vi "Main.vi"() -> ()   [LabVIEW 2020]
uses:
  Ctrl/Ctrl_state_FGV.ctl
panel:
  out "Read Data":u8
  in  "Commande":T1
  out "Compteur 4":dbl
  out "Compteur 3":dbl
  out "Compteur 2":dbl
  out "Compteur":dbl
  # "Non re-entrant"
  # "re-entrant"
  # "FGV"
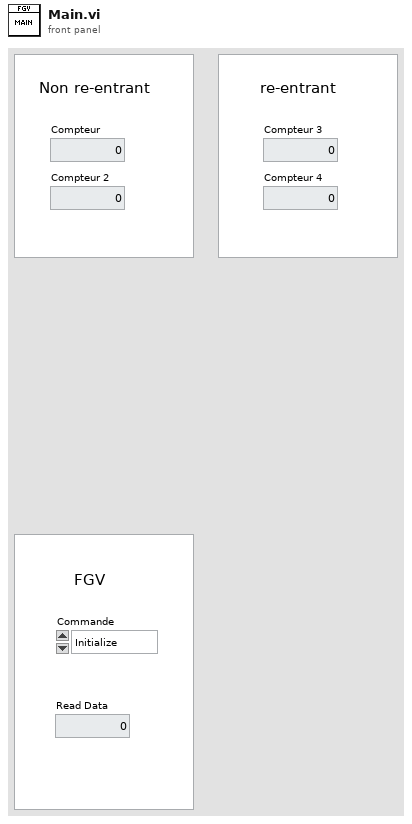
[diagram p1: front panel]
types:
  T1 = typedef "Ctrl_state_FGV.ctl" = enum16{"Initialize", "Write", "Read"}
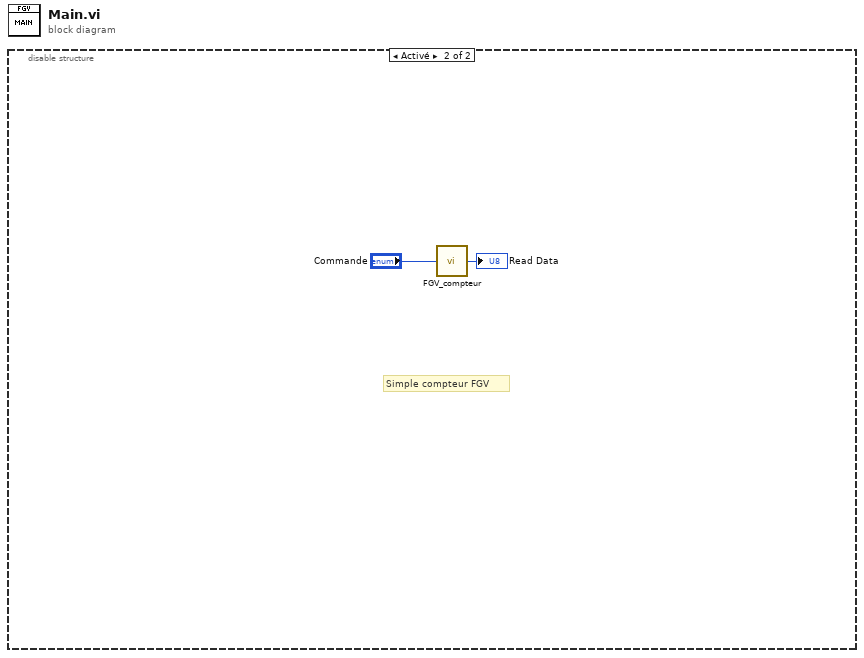
[diagram p0: block diagram]
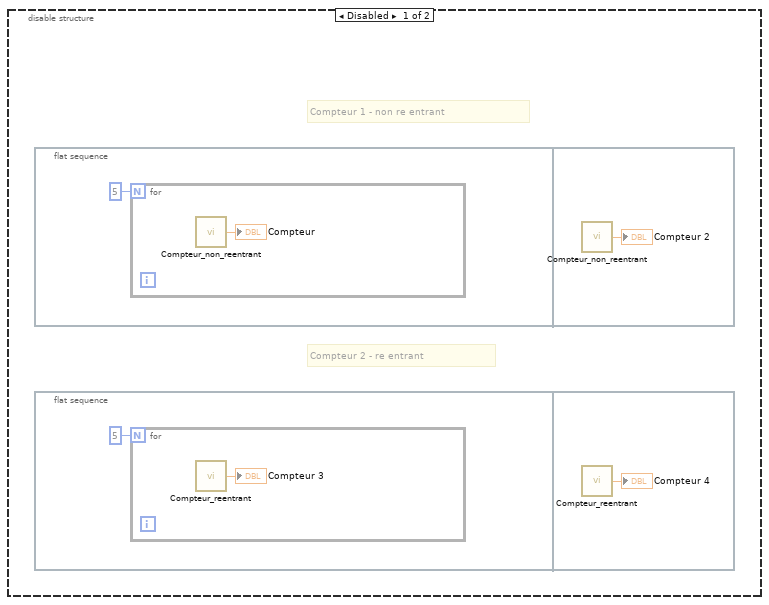
[diagram p2: hidden frame]
diagram:
  n1 = disable-structure shown="Activé" {
    frame Disabled {
      # "Compteur 2 - re entrant"
      # "Compteur 1 - non re entrant"
      n2 = flat-sequence {
        frame #0 {
          n3 = for {
            N: 5 -> [_]
            n4 = call "Compteur_non_reentrant.vi"() -> ("Compteur"=→"Compteur":dbl)  [unwired: 1 in]
          }
        }
        frame #1 {
          n5 = call "Compteur_non_reentrant.vi"() -> ("Compteur"=→"Compteur 2":dbl)  [unwired: 1 in]
        }
      }
      n6 = flat-sequence {
        frame #0 {
          n7 = for {
            N: 5 -> [_]
            n8 = call "Compteur_reentrant.vi"() -> ("Compteur"=→"Compteur 3":dbl)  [unwired: 1 in]
          }
        }
        frame #1 {
          n9 = call "Compteur_reentrant.vi"() -> ("Compteur"=→"Compteur 4":dbl)  [unwired: 1 in]
        }
      }
    }
    frame Enabled {
      # "Simple compteur FGV"
      n10 = call "FGV_compteur.vi"("Commande"="Commande") -> ("Read Data"=→"Read Data":u8)
    }
  }
